vi "getDtXML.vi"(8 "error in (no error)":errorcluster, 11 "ScriptEvent in":refnum<class "ScriptEvent.lvclass">) -> (0 "error out":errorcluster, 2 "dtXML":refnum<class "xmlNode.lvclass">, 3 "ScriptEvent out":refnum<class "ScriptEvent.lvclass">)   [LabVIEW 2009, in "Tools.lvlib" / "Scripting.lvlib" / "ScriptEvent.lvclass"]
uses:
  ScriptEvent.lvclass
  xmlNode/xmlNode.lvclass
  ScriptEvent.lvclass/ScriptEvent.ctl
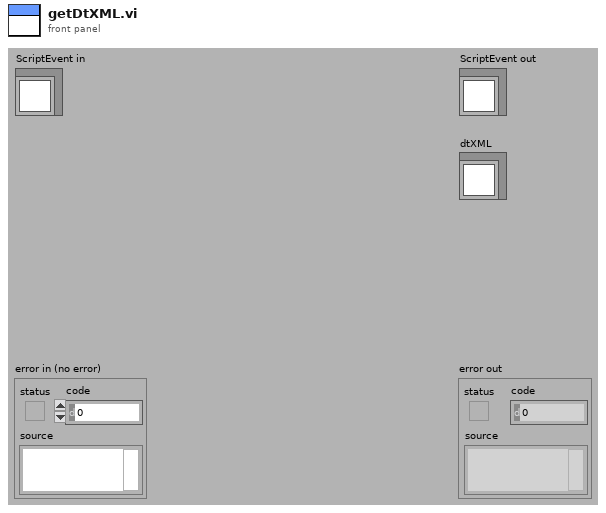
[diagram p1: front panel]
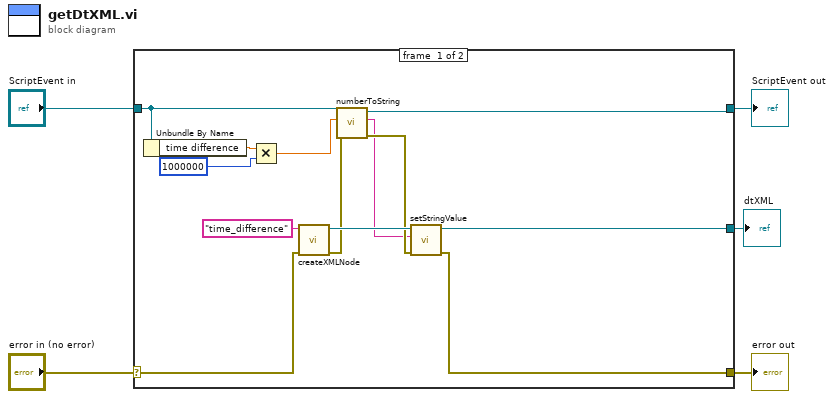
[diagram p0: block diagram]
diagram:
  n1 = case shown="No Error" "error in (no error)" {
    selector: "error in (no error)" -> [w16 w20]
    tunnel: [w15 w20] -> w4
    tunnel: [w6 w19] -> w2
    tunnel: "ScriptEvent in" -> [w11 w19]
    tunnel: [w14 _] -> w1
    frame #0 {
      n2 = Unbundle By Name(w11) -> ("time difference"=w13:dbl)
      n3 = Multiply(x=w13, y=1000000) -> (x*y=w7:dbl)
      n4 = call "createXMLNode.vi"("error in (no error)"=w16, "name"="time_difference") -> ("error out"=w10:errorcluster, "xmlNode out"=w17:refnum<class "xmlNode.lvclass">)  [unwired: 8 in]
      n5 = call "numberToString.vi"("error in (no error)"=w10, "Numeric"=w7, "ScriptEvent in"=w11) -> ("error out"=w9:errorcluster, "String"=w8:string, "ScriptEvent out"=w6:refnum<class "ScriptEvent.lvclass">)  [unwired: 6 in]
      n6 = call-dynamic "setStringValue.vi"("error in (no error)"=w9, "stringValue"=w8, "xmlNode.lvclass in"=w17) -> ("error out"=w15:errorcluster, "xmlNode.lvclass out"=w14:refnum<class "xmlNode.lvclass">)  [unwired: 7 in]
    }
    frame #1 {
    }
  }
  "error out" <- w4
  "ScriptEvent out" <- w2
  "dtXML" <- w1
